vi "Load Inventory.vi"(8 "error in (no error)":errorcluster, 11 "Items in":refnum<class "Items.lvclass">) -> (0 "error out":errorcluster, 3 "Items out":refnum<class "Items.lvclass">)   [LabVIEW 2020, in "Items.lvlib" / "Items.lvclass"]
uses:
  Items.lvclass
  Items.lvclass/Items.ctl
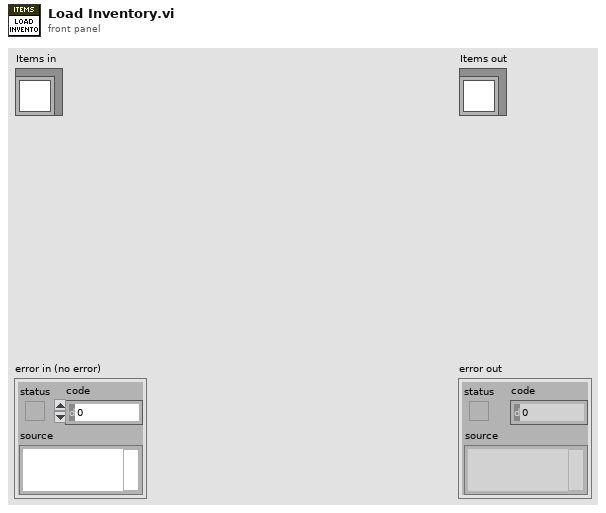
[diagram p1: front panel]
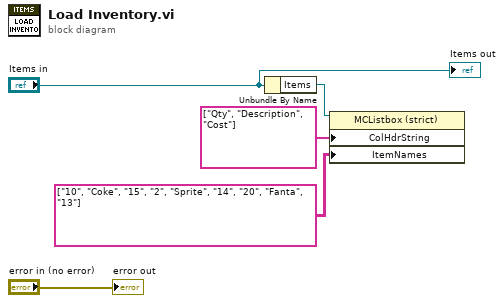
[diagram p0: block diagram]
diagram:
  n1 = Unbundle By Name("Items in") -> ("Items"=w3:refnum<vi>)
  n2 = property class="MCListbox (strict)"(reference=w3, "ColHdrString"=string[] ["Qty", "Description", "Cost"] ("Column Header Strings[]"), "ItemNames"=string[][] [["10", "Coke", "15"], ["2", "Sprite", "14"], ["20", "Fanta", "13"]] ("Item Names")) -> ()  [unwired: 1 in, 2 out]
  "error out" <- "error in (no error)"
  "Items out" <- "Items in"
